vi "Setup UI.vi"(8 "error in (no error)":errorcluster, 10 "Set UI to input? (F)":bool, 11 "Reader in":refnum<class "Reader.lvclass">) -> (0 "error out":errorcluster, 3 "Reader out":refnum<class "Reader.lvclass">)   [LabVIEW 2009, in "Reader.lvclass"]
doc: "Setup UI constructs an object -- populates its member data -- from a front panel the user can see. The VI should be as simple as possible so that a UI loop can poll it continuously for updates. \n\nThe VI is designed to be used as a subPanel within another VI. Wire true to \"Set UI to input\" only on the first call, just after inserting this VI into a subPanel, to populate its controls with the class's current values.\n\nSetup UI is distinct from the class constructor. Class constructors are not polymorphic, yet configure dialogs need to configure objects without knowing their type -- and polymorphism is the necessary solution. Thus, Setup UI is a polymorphic class constructor. This continously polled \"Setup UI\" concept is a kludge: a better idea would be an XControl, but those require a steeper learning curve."
uses:
  Reader.lvclass
  Reader.lvclass/Reader.ctl
  Instruments/Utility Classes/Readable/Readable.lvclass
panel:
  in  "Dwell Time":dbl[unit]
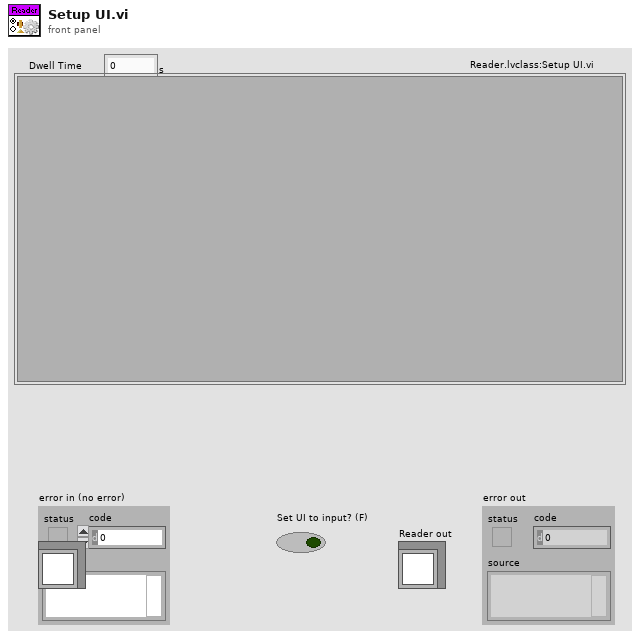
[diagram p1: front panel]
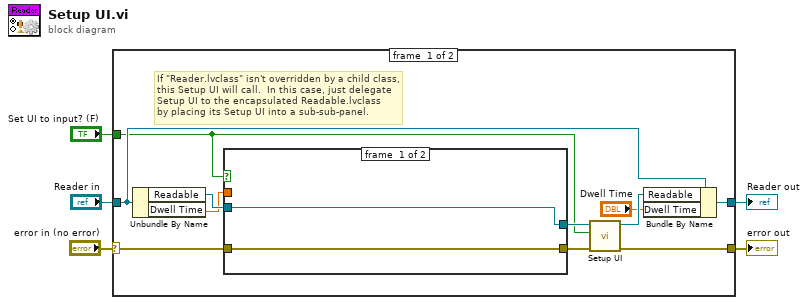
[diagram p0: block diagram]
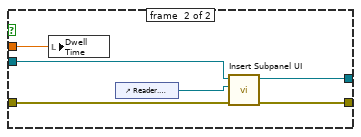
[diagram p2: hidden frame]
diagram:
  n1 = case shown="No Error" "error in (no error)" {
    selector: "error in (no error)" -> [w14 w26]
    tunnel: [w9 w26] -> w4
    tunnel: [w16 w25] -> w1
    tunnel: "Reader in" -> [w13 w25]
    tunnel: "Set UI to input? (F)" -> [w10 _]
    frame #0 {
      # "If \"Reader.lvclass\" isn't overridden by a child class,\nthis Setup UI will call.  In this case, just delegate\nSetup UI to the encapsulated Readable.lvclass\nby placing its Setup UI into a sub-sub-panel."
      n2 = Unbundle By Name(w13) -> ("Readable"=w15:refnum<class "Readable.lvclass">, "Dwell Time"=w6:dbl[unit])
      n3 = case shown="True" w10 {
        tunnel: [w18 w23] -> w11
        tunnel: w15 -> [w18 w22]
        tunnel: w14 -> [w17 w21]
        tunnel: [w17 w20] -> w8
        tunnel: w6 -> [_ w19]
        frame #0 {
        }
        frame #1 {
          n4 = local write "Dwell Time"(w19) -> ()
          n5 = control-ref of="Reader.lvclass:Setup UI.vi"() -> (w24:refnum<vi>)
          n6 = call "Insert Subpanel UI.vi"("error in (no error)"=w21, "Subpanel in"=w24, "LabVIEW Object"=w22) -> ("error out"=w20:errorcluster, "LabVIEW Object out"=w23:refnum<class "Readable.lvclass">)  [unwired: 7 out]
        }
      }
      n7 = call-dynamic "Setup UI.vi"("error in (no error)"=w8, "Set UI to input? (F)"=w10, "Instrument in"=w11) -> ("error out"=w9:errorcluster, "Instrument out"=w12:refnum<class "Readable.lvclass">)  [unwired: 7 out]
      n8 = Bundle By Name(cluster=w13, "Readable"=w12, "Dwell Time"="Dwell Time") -> (w16:refnum<class "Reader.lvclass">)
    }
    frame #1 {
    }
  }
  "error out" <- w4
  "Reader out" <- w1
